vi "190627_FreCTO_kuang.vi"() -> ()   [LabVIEW 2019]
uses:
  <vilib>/rvi/interface/nirviCloseFPGA/nirviCloseFPGA.xnode
  <vilib>/Utility/Variable/NI_VariableUtilities.lvlib
  <vilib>/rvi/interface/nirviReadWriteControl/nirviReadWriteControl.xnode
  <vilib>/rvi/interface/Simulation/niFpgaSimulationCallBeginRW.vi
  <vilib>/rvi/errors/niLvFpgaAdjustHostInterfaceError.vi
  <vilib>/Platform/TimedLoop/XDataNode/XDataNode.xnode
  <vilib>/Platform/TimedLoop/XDataNode/timing_clust.ctl
  <vilib>/Platform/TimedLoop/XDataNode/XDNodeRunTimeDep.lvlib
  <vilib>/Platform/TimedLoop/XDataNode/wakeup.ctl
  <vilib>/Platform/TimedLoop/XDataNode/nitl_modes.ctl
  <vilib>/rvi/interface/nirviMethod/nirviMethod.xnode
  <vilib>/FPGAPlugInAG/Dynamic/niLvFpga_Run_Dynamic.vi
  <vilib>/rvi/interface/nirviOpenFPGA/nirviOpenFPGA.xnode
  <vilib>/FPGAPlugInAG/Dynamic/niLvFpga_Reset_Dynamic.vi
  FPGA_TwoAxisEncoder_revised.vi
  <vilib>/FPGAPlugInAG/Dynamic/niLvFpga_Close_Dynamic.vi
panel:
  in  "Repeat":dbl
  out "Stop by delay":bool
  in  "Debug":bool caption="RUN"
  in  "X_Type":string(combo)="Notch15"
  in  "X_pole":string(combo)="4352"
  in  "Z_Type":string(combo)="Notch15"
  in  "Z_pole":string(combo)="4952"
  out "Time Slots (sec)":dbl[](array[numeric])
  out "All times (sec)":dbl
  out "one period  length":i32
  out "one period start time":i32
  in  "HOST Sample Rate (Hz)":i32=1000
  in  "LOAD":bool
  out "(LS) RMS X (one) (um)":dbl format="%0.4f"
  out "(LS) MAX ERROR X (um)":dbl format="%0.4f"
  out "(LS) RMS ERROR X (um)":dbl format="%0.4f"
  out "(En) RMS X (one) (um)":dbl format="%0.4f"
  out "(LS) RMS Z (one) (um)":dbl format="%0.4f"
  out "(LS) MAX ERROR Z (um)":dbl format="%0.4f"
  out "(LS) RMS ERROR Z (um)":dbl format="%0.4f"
  out "CMD X (rpm)":dbl[](graph)
  out "Linear Scale Position X (mm)":dbl[](graph)
  out "Linear Scale Position Z (mm)":dbl[](graph)
  out "(En) RMS Z (one) (um)":dbl format="%0.4f"
  out "CMD Z (rpm)":dbl[](graph)
  out "Position X (mm)":dbl[](graph)
  out "Linear Scale Position Error X (um)":dbl[](graph)
  out "Linear Scale Position Error Z (um)":dbl[](graph)
  out "Delay":i32
  out "(En) MAX ERROR X (um)":dbl format="%0.4f"
  out "(En) RMS ERROR X (um)":dbl format="%0.4f"
  out "Encoder Position Error X (um)":dbl[](graph)
  out "Position Command X (mm)":dbl[](graph)
  out "(En) MAX ERROR Z (um)":dbl format="%0.4f"
  out "(En) RMS ERROR Z (um)":dbl format="%0.4f"
  out "Encoder Position Error Z (um)":dbl[](graph)
  in  "RUN":bool
  in  "CLEAR":bool
  out "V Loop":bool
  out "Length(Response)":i32
  out "Length(Command)":i32
  out "Done":bool
  out "Error Out (FPGA)":errorcluster
  out "Error Out (Host)":errorcluster
  out "Position Z (mm)":dbl[](graph)
  out "FPGA INITIALIZED":bool
  in  "FPGA Sample Rate (Hz)":dbl=100000.0
  out "Position Command Z (mm)":dbl[](graph)
  in  "STOP":bool
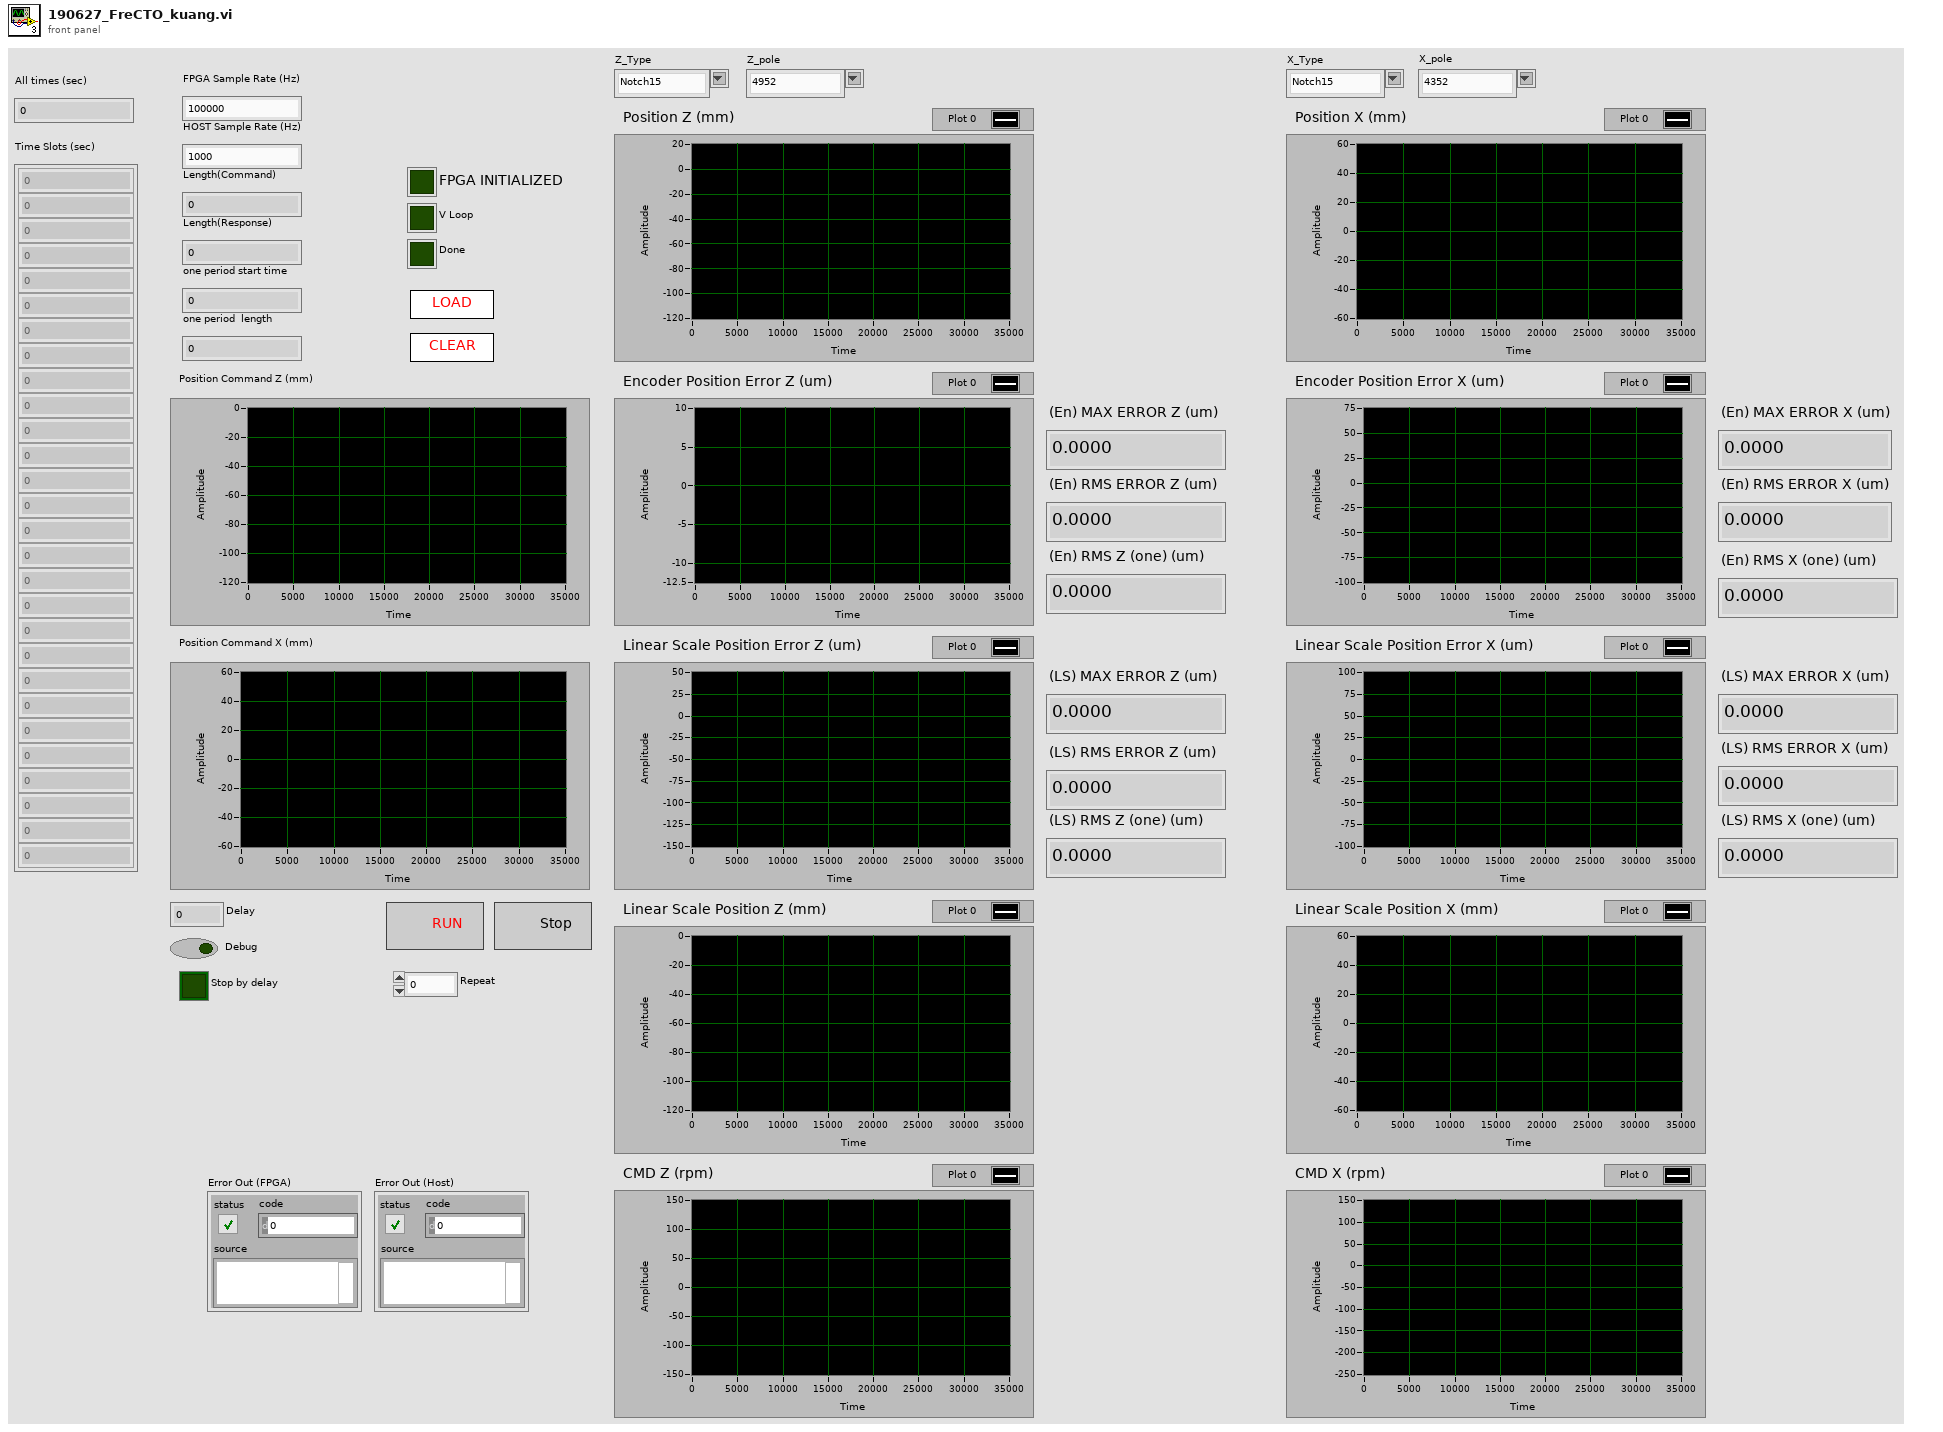
[diagram p1: front panel]
types:
  T1 = typedef "XDNodeRunTimeDep.lvlib/timing_clust.ctl" = cluster{"Expected End [f-1]":u64, "Actual End [f-1]":u64, "Finished Late? [f-1]":bool, "Expected End [i-1]":u64, "Actual End [i-1]":u64, "Finished Late? [i-1]":bool, "Expected Start [i]":u64, "Actual Start [i]":u64, "Expected Start [f]":u64, "Actual Start [f]":u64, "Source Name":string, "Structure Name":string, "Period":i64, "Deadline":i64, "Offset":i64, "Start":i64, "Priority":i32, "Timeout":i32, "Mode":T2, "Wakeup Reason":T3, "Error":errorcluster, "Source Type":string, "Secondary Source Type":string, "Global End Time":u64, "Global Start Time":u64, "Frame Duration":u64, "Iteration Duration":u64, "Assigned CPU":i32, "I/O Scan Engine Mode":u32}
  T2 = typedef "XDNodeRunTimeDep.lvlib/nitl_modes.ctl" = enum32{"No Change", "Process missed periods, maintain original phase", "Discard missed periods, maintain original phase", "Process missed periods, ignore original phase", "Discard missed periods, ignore original phase"}
  T3 = typedef "XDNodeRunTimeDep.lvlib/wakeup.ctl" = enum32{"Normal", "Aborted", "Asynchronous wakeup", "Timing source error", "Timed loop error", "Timeout"}
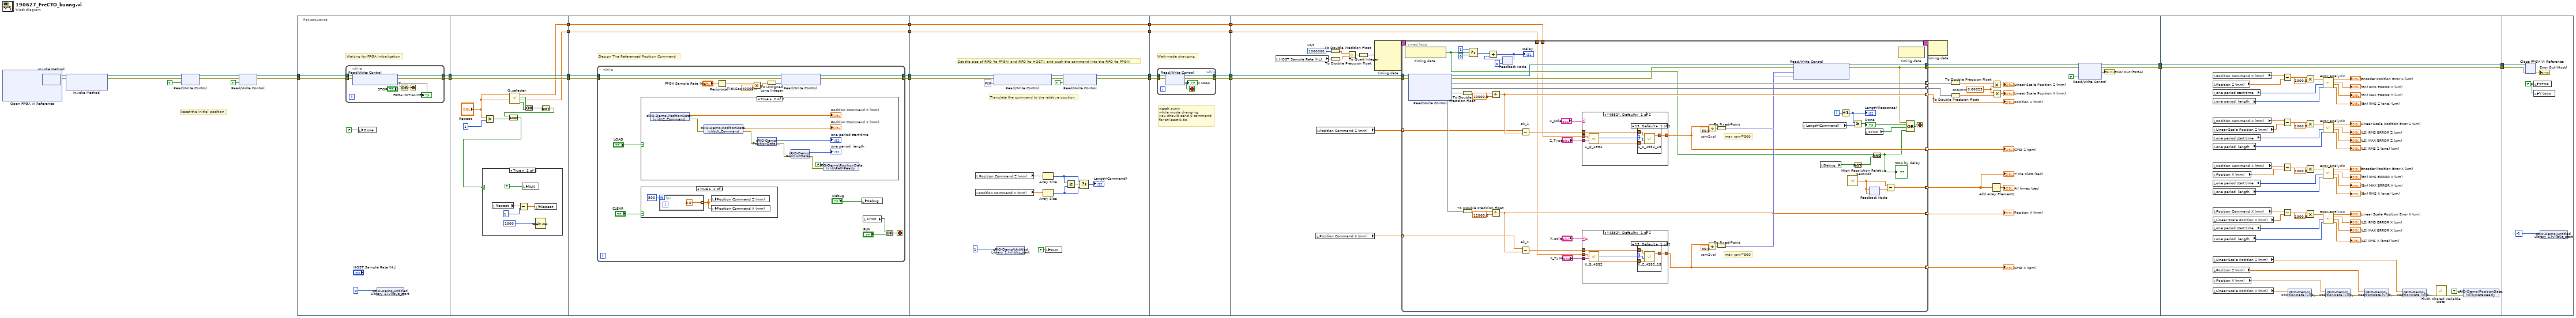
[diagram p0: block diagram]
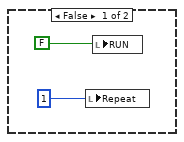
[diagram p2: hidden frame]
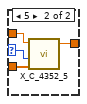
[diagram p5: hidden frame]
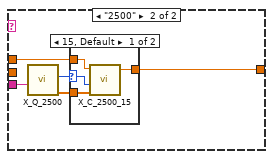
[diagram p6: hidden frame]
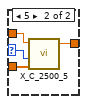
[diagram p7: hidden frame]
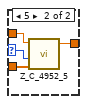
[diagram p8: hidden frame]
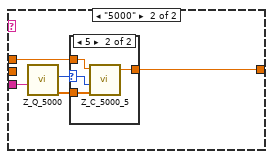
[diagram p9: hidden frame]
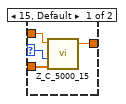
[diagram p10: hidden frame]
diagram:
  # "Reset the initial position"
  n1 = xnode "Open FPGA VI Reference"() -> ("FPGA VI Reference Out"=w17:refnum<k20>, "error out"=w16:errorcluster)  [unwired: 2 in]
  n2 = xnode "Invoke Method"("FPGA VI Reference In"=w17, "error in"=w16) -> ("FPGA VI Reference Out"=w22:refnum<k20>, "error out"=w21:errorcluster)
  n3 = xnode "Invoke Method"("FPGA VI Reference In"=w22, "error in"=w21) -> ("FPGA VI Reference Out"=w15:refnum<k20>, "error out"=w14:errorcluster)  [unwired: 1 in]
  n4 = xnode "Read/Write Control"("FPGA VI Reference In"=w15, "error in"=w14, "Initial"=TRUE ("Reset Encoder")) -> ("FPGA VI Reference Out"=w13:refnum<k20>, "error out"=w12:errorcluster)
  n5 = xnode "Read/Write Control"("FPGA VI Reference In"=w13, "error in"=w12, "Start"=TRUE) -> ("FPGA VI Reference Out"=w20:refnum<k20>, "error out"=w19:errorcluster)
  n6 = flat-sequence {
    tunnel: w20 -> [w40]
    tunnel: w19 -> [w39]
    tunnel: [w38] -> w34
    tunnel: [w37] -> w33
    tunnel: w34 -> [w59]
    tunnel: [w59] -> w10
    tunnel: w33 -> [w58]
    tunnel: [w58] -> w9
    tunnel: [w49] -> w7
    tunnel: [w48] -> w4
    tunnel: [w70] -> w32
    tunnel: [w69] -> w31
    tunnel: w9 -> [w71]
    tunnel: w10 -> [w72]
    tunnel: [w68] -> w8
    tunnel: w7 -> [w68]
    tunnel: w4 -> [w67]
    tunnel: [w67] -> w1
    tunnel: [w115] -> w30
    tunnel: [w114] -> w29
    tunnel: w31 -> [w111]
    tunnel: w32 -> [w112]
    tunnel: w8 -> [w101]
    tunnel: [w101] -> w5
    tunnel: [w100] -> w2
    tunnel: w1 -> [w100]
    tunnel: w30 -> [w121]
    tunnel: [w119] -> w28
    tunnel: w29 -> [w120]
    tunnel: [w118] -> w27
    tunnel: [w117] -> w6
    tunnel: w5 -> [w117]
    tunnel: [w116] -> w3
    tunnel: w2 -> [w116]
    tunnel: w28 -> [w159]
    tunnel: [w156] -> w26
    tunnel: w27 -> [w158]
    tunnel: [w149] -> w25
    tunnel: w6 -> [w128]
    tunnel: w3 -> [w127]
    tunnel: w26 -> [w329]
    tunnel: [w329] -> w24
    tunnel: [w328] -> w23
    tunnel: w25 -> [w328]
    tunnel: w24 -> [w333]
    tunnel: w23 -> [w332]
    frame #0 {
      # "Waiting for FPGA Initialization"
      n7 = while {
        tunnel: w40 -> [w47]
        tunnel: w39 -> [w44]
        tunnel: [w43] -> w37
        tunnel: [w42] -> w38
        stop <- w46 stop-if-true
        n8 = xnode "Read/Write Control"("FPGA VI Reference In"=w47, "error in"=w44) -> ("FPGA VI Reference Out"=w42:refnum<k20>, "error out"=w43:errorcluster, "SYSTEM INITIALIZED"=w41)
        "FPGA INITIALIZED" <- w41
        n9 = Or(x=w41, y="STOP") -> (x .or. y?=w46:bool)
      }
      n10 = local write "Done"(FALSE ("Done")) -> ()
      n11 = shared-variable "cRIO-Demo\\Untitled Library 1.lvlib\\is_start"(0) -> ()  [unwired: 1 in, 1 out]
    }
    frame #1 {
      n12 = Greater?(x="Repeat", y=1) -> (0:w56:bool)
      n13 = call "Q_selecter.vi"("Numeric 5"="Repeat", "Numeric 4"="Repeat") -> ("Boolean 3"=w52:bool, "Array 2"=w48:dbl[], "Boolean 2"=w51:bool, "Array"=w49:dbl[])  [unwired: 6 in]
      n14 = Or(x=w51, y=w52) -> (x .or. y?=w50:bool)
      n15 = Not(x=w50) -> (.not. x?=w55:bool)
      n16 = And(x=w55, y=w56) -> (x .and. y?=w54:bool)
      n17 = case shown="True" w54 {
        frame False {
          n18 = local write "Repeat"(1) -> ()
          n19 = local write "RUN"(FALSE) -> ()
        }
        frame True {
          n20 = local read "Repeat"() -> (w65:dbl)
          n21 = Subtract(x=w65, y=1) -> (x-y=w63:dbl)
          n22 = local write "RUN"(TRUE) -> ()
          n23 = local write "Repeat"(w63) -> ()
          n24 = Wait (ms)(milliseconds to wait=1000) -> ()  [unwired: 1 out]
        }
      }
    }
    frame #2 {
      # "Design The Referenced Position Command"
      n25 = while {
        tunnel: w72 -> [w87]
        tunnel: w71 -> [w86]
        tunnel: [w81] -> w70
        tunnel: [w80] -> w69
        stop <- w79 stop-if-true
        w83 = 40000000.0  # Tick/Sec
        n26 = case shown="True" "LOAD" {
          frame False {
          }
          frame True {
            n27 = shared-variable "cRIO-Demo\\PositionData.lvlib\\Z_Command"() -> (→"Position Command Z (mm)":dbl[], error out=w98:errorcluster)  [unwired: 1 in]
            n28 = shared-variable "cRIO-Demo\\PositionData.lvlib\\X_Command"(error in=w98) -> (→"Position Command X (mm)":dbl[], error out=w94:errorcluster)
            n29 = shared-variable "cRIO-Demo\\PositionData.lvlib\\t0"(error in=w94) -> (→"one period start time":i32, error out=w95:errorcluster)
            n30 = shared-variable "cRIO-Demo\\PositionData.lvlib\\tL"(error in=w95) -> (→"one period  length":i32, error out=w93:errorcluster)
            n31 = shared-variable "cRIO-Demo\\PositionData.lvlib\\PathReady"(FALSE ("PathReady"), error in=w93) -> ()  [unwired: 1 out]
          }
        }
        n32 = case shown="True" "CLEAR" {
          frame False {
          }
          frame True {
            n33 = for {
              N: 500 -> [_]
              tunnel: [0.0 ("element")] -> w89 mode=indexing
            }
            n34 = local write "Position Command Z (mm)"(w89) -> ()
            n35 = local write "Position Command X (mm)"(w89) -> ()
          }
        }
        n36 = Reciprocal(x="FPGA Sample Rate (Hz)") -> (1/x=w84:dbl)
        n37 = Multiply(x=w84, y=w83) -> (x*y=w85:dbl)
        n38 = To Unsigned Long Integer(number=w85) -> (unsigned 32bit integer=w82:u32)
        n39 = xnode "Read/Write Control"("FPGA VI Reference In"=w87, "error in"=w86, "Loop Delay (Tick)"=w82) -> ("FPGA VI Reference Out"=w81:refnum<k20>, "error out"=w80:errorcluster)
        n40 = local write "Debug"("Debug") -> ()
        n41 = local read "STOP"() -> (w78:bool)
        n42 = Or(x=w78, y="RUN") -> (x .or. y?=w79:bool)
      }
    }
    frame #3 {
      # "Translate the command to the relative position"
      # "Set the size of FIFO (to FPGA) and FIFO (to HOST), and push the command into the FIFO (to FPGA)"
      n43 = local read "Position Command X (mm)"() -> (w104:dbl[])
      n44 = local read "Position Command Z (mm)"() -> (w105:dbl[])
      n45 = xnode "Read/Write Control"("FPGA VI Reference In"=w112, "Output Votage Bound (vol)"=fxp<+,20,5> 10.0) -> ()  [unwired: 1 in, 2 out]
      n46 = shared-variable "cRIO-Demo\\Untitled Library 1.lvlib\\is_start"(1) -> ()  [unwired: 1 in, 1 out]
      n47 = Array Size(array=w105) -> (size(s)=w108:i32)
      n48 = Array Size(array=w104) -> (size(s)=w107:i32)
      n49 = local write "RUN"(FALSE) -> ()
      n50 = xnode "Read/Write Control"("FPGA VI Reference In"=w112, "error in"=w111, "HOST READY?"=TRUE) -> ("FPGA VI Reference Out"=w115:refnum<k20>, "error out"=w114:errorcluster)
      n51 = Greater Or Equal?(x=w108, y=w107) -> (x >= y?=w109:bool)
      n52 = Select(t=w108, s=w109, f=w107) -> (s? t:f=→"Length(Command)":i32)
    }
    frame #4 {
      # "watch out!!!\nwhile mode changing\nyou should send 0 command\nfor at least 0.5s."
      # "Wait mode changing"
      n53 = while {
        tunnel: w121 -> [w126]
        tunnel: w120 -> [w125]
        tunnel: [w124] -> w119
        tunnel: [w123] -> w118
        stop <- w122 stop-if-true
        n54 = xnode "Read/Write Control"("FPGA VI Reference In"=w126, "error in"=w125) -> ("FPGA VI Reference Out"=w124:refnum<k20>, "error out"=w123:errorcluster, "V Loop"=w122)
        "V Loop" <- w122
      }
    }
    frame #5 {
      w131 = 0.00025  # cnt2mm
      w153 = 1000000  # us/s
      n55 = local read "HOST Sample Rate (Hz)"() -> (w142:i32)
      n56 = local read "Position Command X (mm)"() -> (w140:dbl[])
      n57 = local read "Position Command Z (mm)"() -> (w141:dbl[])
      n58 = To Double Precision Float(number=w153) -> (double precision float=w145:dbl)
      n59 = To Double Precision Float(number=w142) -> (double precision float=w146:dbl)
      n60 = Divide(x=w145, y=w146) -> (x/y=w152:dbl)
      n61 = To Quad Integer(1:w152) -> (0:w151:i64)
      n62 = node-c288(w151) -> (w155:T1)  [unwired: 3 in]
      n63 = timed-loop {
        tunnel: w159 -> [w198]
        tunnel: w158 -> [w196]
        tunnel: [w182] -> w157
        timing: w155 -> [_]
        timing-out: [_] -> w154
        tunnel: [w181] -> w150
        tunnel: [w192] -> w136 mode=indexing
        tunnel: [w189] -> w134 mode=indexing
        tunnel: [w167] -> w143 mode=indexing
        tunnel: [w193] -> w135 mode=indexing
        tunnel: w141 -> [w176] mode=indexing
        tunnel: w140 -> [w175] mode=indexing
        tunnel: [w168] -> w139 mode=indexing
        tunnel: [w187] -> w133 mode=indexing
        tunnel: [w177] -> w129 mode=indexing
        tunnel: w128 -> [w161]
        tunnel: w127 -> [w160]
        i -> [w207]
        stop <- w212 stop-if-true
        w191 = 30.0  # rpm2vol
        w208 = 30.0  # rpm2vol
        # "max rpm=300"
        # "max rpm=300"
        n64 = node-c288() -> (w163:bool)  [unwired: 1 in]
        n65 = xnode "Read/Write Control"("FPGA VI Reference In"=w198, "error in"=w196) -> ("FPGA VI Reference Out"=w186:refnum<k20>, "error out"=w185:errorcluster, "Line Scale Z (count)"=w189, "Line Scale X (count)"=w187, "Encoder Z (count)"=w188, "Encoder X (count)"=w180)
        n66 = To Double Precision Float(number=w188) -> (double precision float=w206:dbl)
        n67 = To Double Precision Float(number=w180) -> (double precision float=w195:dbl)
        n68 = Select(t=1, s=w163, f=0) -> (s? t:f=w201:i32)
        n69 = Divide(x=w206, y=10000.0) -> (x/y=w192:dbl)
        n70 = Divide(x=w195, y=12000.0) -> (x/y=w193:dbl)
        n71 = feedback #1(0) -> (w200:i32)
        n72 = Add(x=w201, y=w200) -> (x+y=w162:i32)
        "Delay" <- w162
        n73 = feedback-in #1(w162) -> ()
        n74 = Subtract "ek_Z"(x=w176, y=w192) -> (x-y=w172:dbl)
        n75 = Subtract "ek_X"(x=w175, y=w193) -> (x-y=w169:dbl)
        n76 = case shown="\"4952\", Default" "Z_pole" {
          tunnel: "Z_Type" -> [w245 w258]
          tunnel: w172 -> [w243 w255]
          tunnel: [w242 w254] -> w167
          tunnel: w161 -> [w240 _]
          frame "4952", Default {
            n77 = call "Z_Q_4952.vi"("Type"=w245, "Qn 2"=w240) -> ("Qn"=w241:dbl[], "L"=w244:i32)  [unwired: 8 in]
            n78 = case shown="15, Default" w244 {
              selector: w244 -> [w247 w251]
              tunnel: w241 -> [w246 w250]
              tunnel: w243 -> [w249 w253]
              tunnel: [w248 w252] -> w242
              frame 15, Default {
                n79 = call "Z_C_4952_15.vi"("ek"=w249, "length"=w247, "q"=w246) -> ("uk"=w248:dbl)  [unwired: 4 in]
              }
              frame 5 {
                n80 = call "Z_C_4952_5.vi"("ek"=w253, "length"=w251, "q"=w250) -> ("uk"=w252:dbl)  [unwired: 4 in]
              }
            }
          }
          frame "5000" {
            n81 = call "Z_Q_5000.vi"("Type"=w258) -> ("Qn"=w256:dbl[], "L"=w257:i32)  [unwired: 9 in]
            n82 = case shown="5" w257 {
              selector: w257 -> [w260 w264]
              tunnel: w256 -> [w259 w263]
              tunnel: w255 -> [w262 w266]
              tunnel: [w261 w265] -> w254
              frame 15, Default {
                n83 = call "Z_C_5000_15.vi"("ek"=w262, "length"=w260, "q"=w259) -> ("uk"=w261:dbl)  [unwired: 4 in]
              }
              frame 5 {
                n84 = call "Z_C_5000_5.vi"("ek"=w266, "length"=w264, "q"=w263) -> ("uk"=w265:dbl)  [unwired: 4 in]
              }
            }
          }
        }
        n85 = case shown="\"4352\", Default" "X_pole" {
          tunnel: "X_Type" -> [w218 w231]
          tunnel: w169 -> [w216 w228]
          tunnel: [w215 w227] -> w168
          tunnel: w160 -> [w213 _]
          frame "4352", Default {
            n86 = call "X_Q_4352.vi"("Type"=w218, "Qn 2"=w213) -> ("Qn"=w214:dbl[], "L"=w217:i32)  [unwired: 8 in]
            n87 = case shown="15, Default" w217 {
              selector: w217 -> [w220 w224]
              tunnel: w214 -> [w219 w223]
              tunnel: w216 -> [w222 w226]
              tunnel: [w221 w225] -> w215
              frame 15, Default {
                n88 = call "X_C_4352_15.vi"("ek"=w222, "length"=w220, "q"=w219) -> ("uk"=w221:dbl)  [unwired: 4 in]
              }
              frame 5 {
                n89 = call "X_C_4352_5.vi"("ek"=w226, "length"=w224, "q"=w223) -> ("uk"=w225:dbl)  [unwired: 4 in]
              }
            }
          }
          frame "2500" {
            n90 = call "X_Q_2500.vi"("Type"=w231) -> ("Qn"=w229:dbl[], "L"=w230:i32)  [unwired: 9 in]
            n91 = case shown="15, Default" w230 {
              selector: w230 -> [w233 w237]
              tunnel: w229 -> [w232 w236]
              tunnel: w228 -> [w235 w239]
              tunnel: [w234 w238] -> w227
              frame 15, Default {
                n92 = call "X_C_2500_15.vi"("ek"=w235, "length"=w233, "q"=w232) -> ("uk"=w234:dbl)  [unwired: 4 in]
              }
              frame 5 {
                n93 = call "X_C_2500_5.vi"("ek"=w239, "length"=w237, "q"=w236) -> ("uk"=w238:dbl)  [unwired: 4 in]
              }
            }
          }
        }
        n94 = Divide(x=w167, y=w208) -> (x/y=w209:fxp<+/-,20,5>)
        n95 = Divide(x=w168, y=w191) -> (x/y=w190:fxp<+/-,20,5>)
        n96 = To Fixed-Point(number=w209) -> (fixed-point=w184:fxp<+/-,20,5>)  [unwired: 1 in]
        n97 = To Fixed-Point(number=w190) -> (fixed-point=w183:fxp<+/-,20,5>)  [unwired: 1 in]
        n98 = xnode "Read/Write Control"("FPGA VI Reference In"=w186, "error in"=w185, "Velocity Command Z (vol)"=w184, "Velocity Command X (vol)"=w183) -> ("FPGA VI Reference Out"=w182:refnum<k20>, "error out"=w181:errorcluster)
        n99 = local read "Length(Command)"() -> (w197:i32)
        n100 = local read "Debug"() -> (w166:bool)
        n101 = Increment(x=w207) -> (x+1=w204:i32)
        "Length(Response)" <- w204
        n102 = call <vilib>:"High Resolution Relative Seconds.vi"() -> ("relative seconds"=w179:dbl)
        n103 = Greater Or Equal?(x=w204, y=w197) -> (x >= y?=w211:bool)
        "Done" <- w211
        n104 = Not(x=w166) -> (.not. x?=w165:bool)
        n105 = local read "STOP"() -> (w210:bool)
        n106 = feedback #2(w179) -> (w178:dbl)
        n107 = feedback-in #2(w179) -> ()
        n108 = And(x=w163, y=w165) -> (x .and. y?=w164:bool)
        "Stop by delay" <- w164
        n109 = Subtract(x=w179, y=w178) -> (x-y=w177:dbl)
        n110 = node-c288() -> ()  [unwired: 1 in, 1 out]
        n111 = Compound Arithmetic op=OR(w181, w211, w210, w164) -> (w212:bool)
      }
      "Position Z (mm)" <- w136
      "Position X (mm)" <- w135
      "CMD Z (rpm)" <- w143
      "CMD X (rpm)" <- w139
      "Time Slots (sec)" <- w129
      n112 = node-c288(w154) -> ()  [unwired: 1 out]
      n113 = To Double Precision Float(number=w134) -> (double precision float=w132:dbl[])
      n114 = To Double Precision Float(number=w133) -> (double precision float=w138:dbl[])
      n115 = Add Array Elements(numeric array=w129) -> (sum=→"All times (sec)":dbl)
      n116 = Multiply(x=w132, y=w131) -> (x*y=→"Linear Scale Position Z (mm)":dbl[])
      n117 = Multiply(x=w131, y=w138) -> (x*y=→"Linear Scale Position X (mm)":dbl[])
      n118 = xnode "Read/Write Control"("FPGA VI Reference In"=w157, "error in"=w150, "stop"=TRUE) -> ("FPGA VI Reference Out"=w156:refnum<k20>, "error out"=w149:errorcluster, "Error Out"=→"Error Out (FPGA)")
    }
    frame #6 {
      n119 = local read "Position Command Z (mm)"() -> (w327:dbl[])
      n120 = local read "Position Z (mm)"() -> (w326:dbl[])
      n121 = local read "one period start time"() -> (w317:i32)
      n122 = local read "one period  length"() -> (w316:i32)
      n123 = local read "Position Command Z (mm)"() -> (w280:dbl[])
      n124 = local read "Linear Scale Position Z (mm)"() -> (w323:dbl[])
      n125 = local read "one period start time"() -> (w311:i32)
      n126 = local read "one period  length"() -> (w310:i32)
      n127 = local read "Position Command X (mm)"() -> (w298:dbl[])
      n128 = local read "Position X (mm)"() -> (w297:dbl[])
      n129 = local read "one period start time"() -> (w296:i32)
      n130 = local read "one period  length"() -> (w295:i32)
      n131 = local read "Position Command X (mm)"() -> (w281:dbl[])
      n132 = local read "Linear Scale Position X (mm)"() -> (w294:dbl[])
      n133 = local read "one period start time"() -> (w293:i32)
      n134 = local read "one period  length"() -> (w292:i32)
      n135 = local read "Linear Scale Position Z (mm)"() -> (w290:dbl[])
      n136 = local read "Position Z (mm)"() -> (w282:dbl[])
      n137 = local read "Position X (mm)"() -> (w283:dbl[])
      n138 = local read "Linear Scale Position X (mm)"() -> (w291:dbl[])
      n139 = Subtract(x=w327, y=w326) -> (x-y=w324:dbl[])
      n140 = Subtract(x=w280, y=w323) -> (x-y=w275:dbl[])
      n141 = Subtract(x=w298, y=w297) -> (x-y=w308:dbl[])
      n142 = Subtract(x=w281, y=w294) -> (x-y=w279:dbl[])
      n143 = shared-variable "cRIO-Demo\\PositionData.lvlib\\X_LS"(w291) -> (error out=w289:errorcluster)  [unwired: 1 in]
      n144 = Multiply(x=w324, y=1000.0) -> (x*y=w322:dbl[])
      n145 = Multiply(x=w275, y=1000.0) -> (x*y=w274:dbl[])
      n146 = Multiply(x=w308, y=1000.0) -> (x*y=w309:dbl[])
      n147 = Multiply(x=w279, y=1000.0) -> (x*y=w277:dbl[])
      n148 = call "error_analysis.vi"("tLength"=w316, "t0"=w317, "data in (um)"=w322) -> ("rms (one) (um)"=→"(En) RMS Z (one) (um)":dbl, "max err (um)"=→"(En) MAX ERROR Z (um)":dbl, "rms (all) (um)"=→"(En) RMS ERROR Z (um)":dbl, "data out (um)"=→"Encoder Position Error Z (um)":dbl[])  [unwired: 5 in]
      n149 = call "error_analysis.vi"("tLength"=w310, "t0"=w311, "data in (um)"=w274) -> ("rms (one) (um)"=→"(LS) RMS Z (one) (um)":dbl, "max err (um)"=→"(LS) MAX ERROR Z (um)":dbl, "rms (all) (um)"=→"(LS) RMS ERROR Z (um)":dbl, "data out (um)"=→"Linear Scale Position Error Z (um)":dbl[])  [unwired: 5 in]
      n150 = call "error_analysis.vi"("tLength"=w295, "t0"=w296, "data in (um)"=w309) -> ("rms (one) (um)"=→"(En) RMS X (one) (um)":dbl, "max err (um)"=→"(En) MAX ERROR X (um)":dbl, "rms (all) (um)"=→"(En) RMS ERROR X (um)":dbl, "data out (um)"=→"Encoder Position Error X (um)":dbl[])  [unwired: 5 in]
      n151 = call "error_analysis.vi"("tLength"=w292, "t0"=w293, "data in (um)"=w277) -> ("rms (one) (um)"=→"(LS) RMS X (one) (um)":dbl, "max err (um)"=→"(LS) MAX ERROR X (um)":dbl, "rms (all) (um)"=→"(LS) RMS ERROR X (um)":dbl, "data out (um)"=→"Linear Scale Position Error X (um)":dbl[])  [unwired: 5 in]
      n152 = shared-variable "cRIO-Demo\\PositionData.lvlib\\X_EN"(w283, error in=w289) -> (error out=w288:errorcluster)
      n153 = shared-variable "cRIO-Demo\\PositionData.lvlib\\Z_EN"(w282, error in=w288) -> (error out=w287:errorcluster)
      n154 = shared-variable "cRIO-Demo\\PositionData.lvlib\\Z_LS"(w290, error in=w287) -> (error out=w286:errorcluster)
      n155 = call <vilib>:"Flush Shared Variable Data.vi"("error in (no error)"=w286) -> ("error out"=w285:errorcluster)  [unwired: 10 in]
      n156 = shared-variable "cRIO-Demo\\PositionData.lvlib\\DataReady"(TRUE, error in=w285) -> ()  [unwired: 1 out]
    }
    frame #7 {
      w331 = FALSE ("STOP")
      n157 = xnode "Close FPGA VI Reference"("FPGA VI Reference In"=w333, "error in"=w332) -> ("error out"=→"Error Out (Host)":errorcluster)
      n158 = local write "STOP"(w331) -> ()
      n159 = local write "V Loop"(w331) -> ()
      n160 = shared-variable "cRIO-Demo\\Untitled Library 1.lvlib\\is_start"(-1) -> ()  [unwired: 1 in, 1 out]
    }
  }
